vi "Log Regex Checker.vi"(7 "Log String":string, 8 "error in":errorcluster, 9 "Expected Log Text (Any)":string, 10 "Expected Log Level (Any)":string, 11 "Expected Logger Name (Any)":string) -> (0 "error out":errorcluster, 2 "whole match":string, 3 "Math Found":bool)   [LabVIEW 2020]
uses:
  <vilib>/regexp/Match Regular Expression.xnode
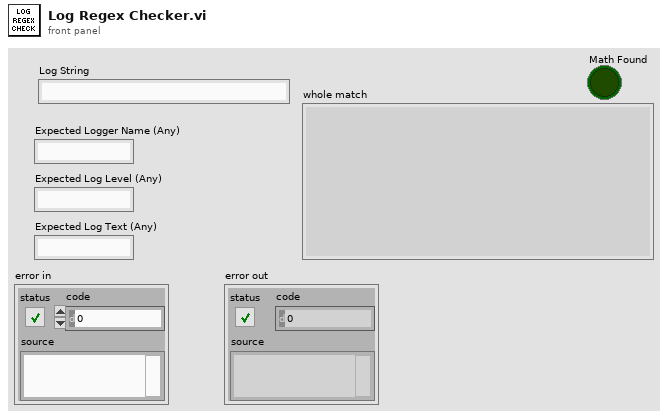
[diagram p1: front panel]
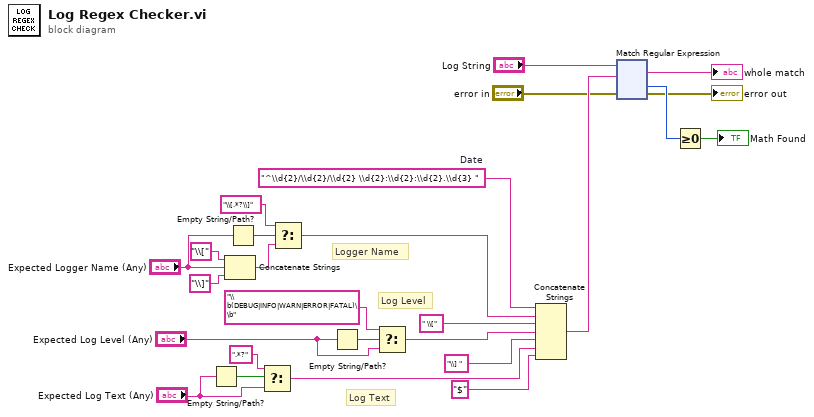
[diagram p0: block diagram]
diagram:
  w25 = "^\\d{2}/\\d{2}/\\d{2} \\d{2}:\\d{2}:\\d{2}.\\d{3} "  # Date
  # "Log Level"
  # "Log Text"
  # "Logger Name"
  n1 = Empty String/Path?(string/path="Expected Log Text (Any)") -> (empty?=w6:bool)
  n2 = Concatenate Strings("\\[" ("f"), "Expected Logger Name (Any)", "\\]" ("f")) -> (w7:string)
  n3 = Empty String/Path?(string/path="Expected Logger Name (Any)") -> (empty?=w13:bool)
  n4 = Select(t=".*?", s=w6, f="Expected Log Text (Any)") -> (s? t:f=w5:string)
  n5 = Select(t="\\[.*?\\]", s=w13, f=w7) -> (s? t:f=w12:string)
  n6 = Empty String/Path?(string/path="Expected Log Level (Any)") -> (empty?=w16:bool)
  n7 = Select(t="\\b(DEBUG|INFO|WARN|ERROR|FATAL)\\b", s=w16, f="Expected Log Level (Any)") -> (s? t:f=w14:string)
  n8 = Concatenate Strings(w25, w12, " \\[", w14, "\\] ", w5, "$" ("string")) -> (w22:string)
  n9 = xnode "Match Regular Expression"("input string"="Log String", "regular expression"=w22, "error in"="error in") -> ("whole match"=→"whole match":string, "offset past match"=w21:i32, "error out"=→"error out":errorcluster)  [unwired: 3 in, 2 out]
  n10 = Greater Or Equal To 0?(x=w21) -> (x >= 0?=→"Math Found":bool)
